vi "Hydrodynamics Method_YCC.vi"(11 "Save?":bool) -> ()   [LabVIEW 2014]
uses:
  <vilib>/Analysis/3filter.llb/Savitzky-Golay Filter (DBL).vi
  <vilib>/DAQmx/create/channels.llb/DAQmx Create Channel (AI-Voltage-Basic).vi
  <vilib>/DAQmx/configure/timing.llb/DAQmx Timing (Sample Clock).vi
  <vilib>/DAQmx/read.llb/DAQmx Read (Analog 1D DBL 1Chan NSamp).vi
  <vilib>/gmath/NumericalOptimization/Nonlinear Curve Fit LM formula string.vi
  Main-Stage-PI/(Global) Current handle and LaserPower_YCC.vi
  <vilib>/Analysis/NI_AALBase.lvlib
  <vilib>/gmath/NI_Gmath.lvlib
panel:
  out "Filtered data":dbl[](array[numeric])
  in  "Who's Data":enum16{"YCC", "PYW", "LCH", "YYH"}(ring)
  in  "Custum Fs (Hz)":i32
  in  "Sampling Rate Enum (Hz)":T1(ring)=enum."131072"
  out "output array":dbl[](array[numeric])
  in  "Filter?":bool=TRUE
  in  "add record time (s)":dbl
  out "data":dbl[](array[numeric])
  out "lower peak (mV)":dbl
  out "upper peak (mV)":dbl
  out "middle peak (mV)":dbl
  in  "Volumn of glycerol":dbl
  in  "Volumn of water":dbl=1.0
  in  "Temperature (C)":dbl=25.0
  out "best fit parameters":dbl[](array[numeric])
  out "best nonlinear fit counts":dbl[](array[numeric])
  out "QPD (1000X V)":dbl[](array[numeric])
  out "Normalized Counts":dbl[](array[numeric])
  out "dx (nm)":dbl
  out "Histogram: h(x)":i32[](array[numeric])
  in  "Cut second from initial":dbl
  in  "side points":i32=32
  out "Axis":i32
  in  "MultiGaussian Fit?":bool=TRUE
  out "Wait between half period (s)":dbl=0.2
  out "Real Current Commanded position (um)":dbl format="%0.5f"
  out "Trap stiffness (pN/nm)":dbl
  out "Drag Force (pN)":dbl
  out "Conversion factor (V/um)":dbl=1.5
  out "dx (V)":dbl
  out "dx2 (mV)":dbl
  out "dx1 (mV)":dbl
  in  "bead height (um)":dbl=2.0
  out "Upper QPD":dbl
  out "Lower QPD":dbl
  out "Center QPD":dbl
  out "Time":dbl[](array[numeric])
  in  "Tab Control":T2(tab)
  out "Raw XY Graph":cluster{dbl[], "data":dbl[]}(graph)
  out "Filtered XY Graph":cluster{dbl[], "Filtered X":dbl[]}(graph)
  out "Histogram Graph":T3(graph)
  out "XY Graph":T4(graph)
  out "Sampling rate (Hz)":dbl=32000.0 format="%0.2f"
  out "traveling time (s)":dbl
  out "True rate?":bool
  in  "T=X\nF=Y":bool=TRUE
  in  "T= + first\nF=- first":bool
  in  "range  (um)":dbl=10.0 min=0.0 max=100.0 step=0.5 format="%.3f"
  in  "scan rate  (um/s)":dbl=200.0 format="%.3f"
  in  "# of period generate\n(0.5,1,1.5,2...)":dbl=4.0
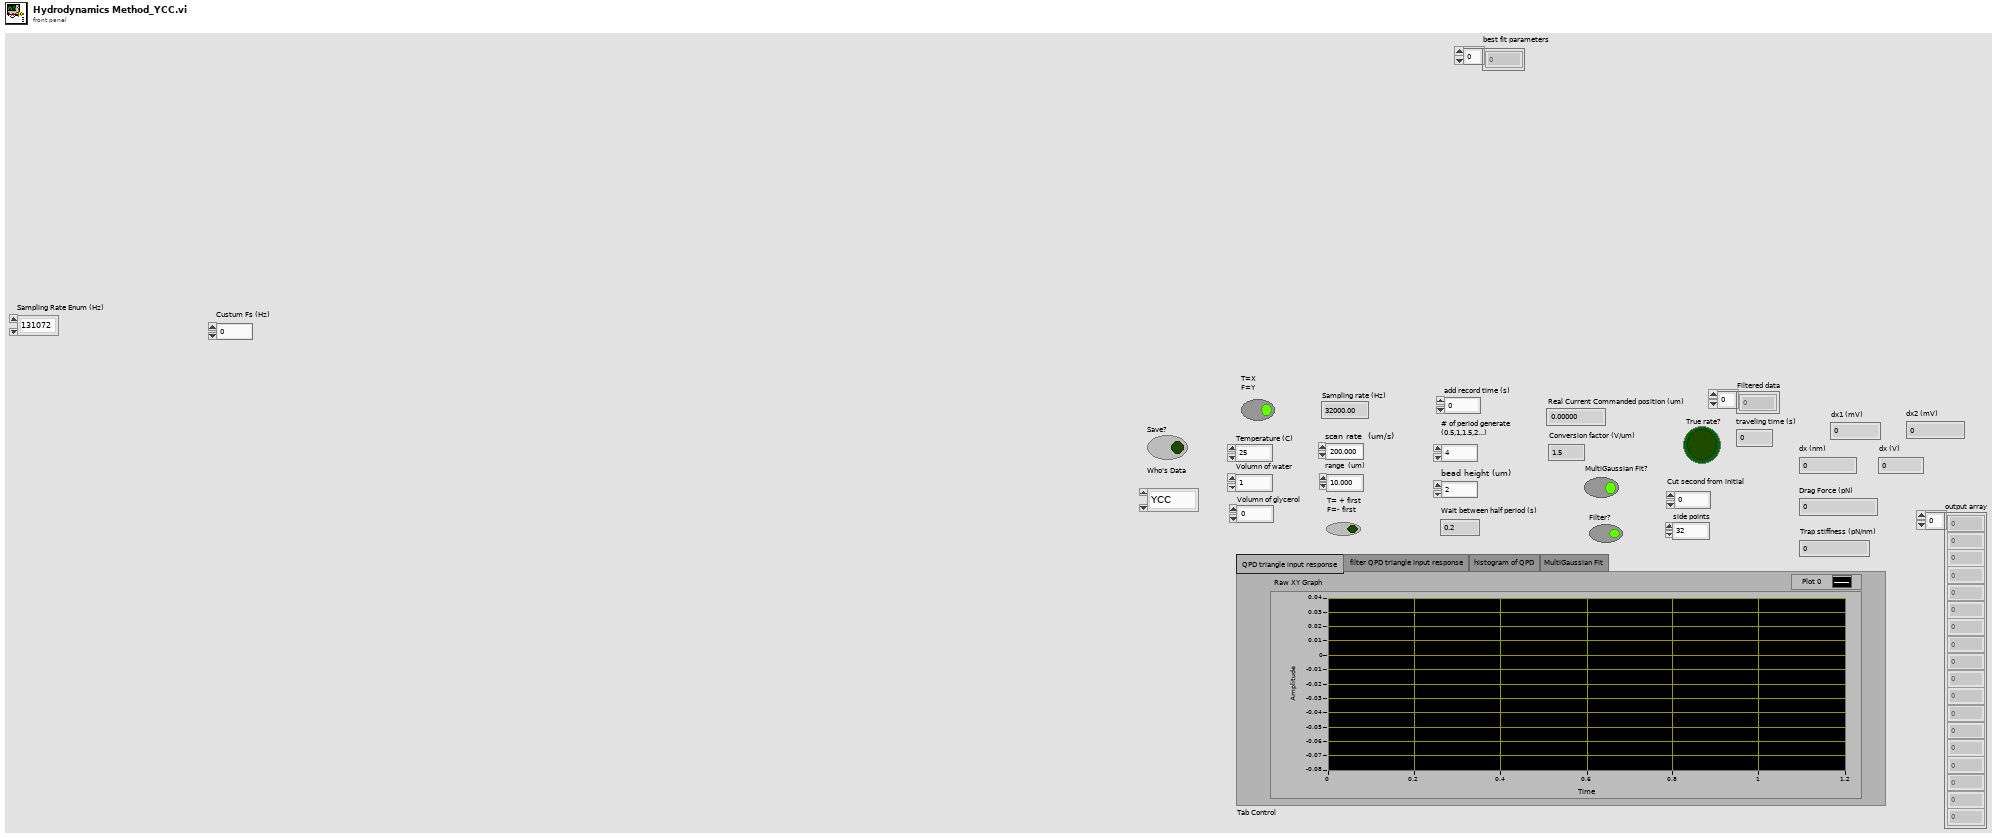
[diagram p1: front panel]
types:
  T1 = enum16{"custum", "16384", "32768", "65536", "131072", "262144"}
  T2 = enum32{"QPD triangle input response ", "filter QPD triangle input response ", "histogram of QPD", "MultiGaussian Fit"}
  T3 = cluster{"X Values":dbl[], "Histogram: h(x)":i32[]}
  T4 = cluster{"QPD (1000X V)":dbl[], "Nor. Counts":dbl[]}[]
  T5 = cluster{"model":string, "Parameters":string[], "x":string}
  T6 = cluster{"QPD (1000X V)":dbl[], "best nonlinear fit counts":dbl[]}
  T7 = cluster{"QPD (1000X V)":dbl[], "Normalized Counts":dbl[]}
  T8 = cluster{"QPD (1000X V)":dbl[], "Normalized Counts":dbl[]}[]
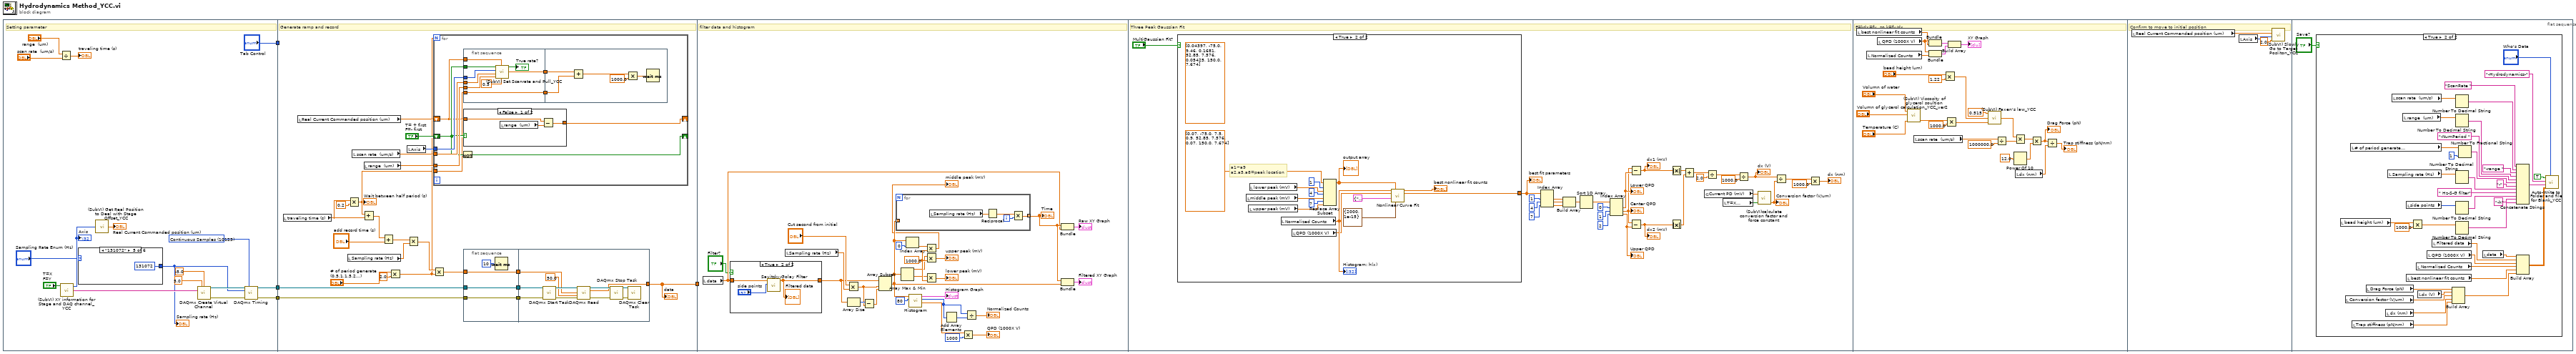
[diagram p0: block diagram]
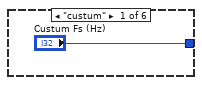
[diagram p2: hidden frame]
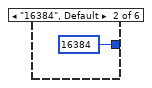
[diagram p3: hidden frame]
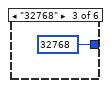
[diagram p4: hidden frame]
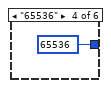
[diagram p5: hidden frame]
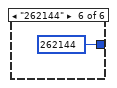
[diagram p6: hidden frame]
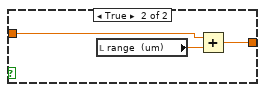
[diagram p7: hidden frame]
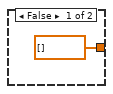
[diagram p9: hidden frame]
diagram:
  n1 = flat-sequence {
    tunnel: ["Tab Control"] -> w4
    tunnel: [w8] -> w2
    tunnel: [w7] -> w1
    tunnel: w4 -> [_]
    tunnel: [w39] -> w3
    tunnel: w2 -> [w43]
    tunnel: w1 -> [w42]
    tunnel: w3 -> [_]
    frame #0 {
      w21 = 10123 items=["Finite Samples"=10178, "Continuous Samples"=10123, "Hardware Timed Single Point"=12522] ("sample mode")
      # "Setting parameter"
      n2 = Divide(x="range  (um)", y="scan rate  (um/s)") -> (x/y=→"traveling time (s)":dbl)
      n3 = call "(SubVI) XY information for Stage and DAQ channel_YCC.vi"("T=X\nF=Y"="T=X\nF=Y") -> ("physical channels"=w17:tag, "Axis"=w10:i32)  [unwired: 3 in]
      "Axis" <- w10
      n4 = case shown="\"131072\"" "Sampling Rate Enum (Hz)" {
        tunnel: ["Custum Fs (Hz)" 16384 32768 65536 131072 262144] -> w5
        frame "custum" {
        }
        frame "16384", Default {
        }
        frame "32768" {
        }
        frame "65536" {
        }
        frame "131072" {
        }
        frame "262144" {
        }
      }
      "Sampling rate (Hz)" <- w5
      n5 = call "(SubVI) Get Real Position to Deal with Stage Offset_YCC.vi"("Axis"=w10) -> ("Real Current Commanded position (um)"=→"Real Current Commanded position (um)":dbl)  [unwired: 3 in, 1 out]
      n6 = call-poly <vilib>:"DAQmx Create Virtual Channel.vi"("maximum value"=5.0, "minimum value"=-5.0, "physical channels"=w17) -> ("task out"=w19:refnum<k21>, "error out"=w20:errorcluster)  [unwired: 6 in, 5 out]
      n7 = call-poly <vilib>:"DAQmx Timing.vi"("task/channels in"=w19, "sample mode"=w21, "rate"=w5, "error in"=w20) -> ("task out"=w8:refnum<k21>, "error out"=w7:errorcluster)  [unwired: 3 in, 7 out]
    }
    frame #1 {
      # "Generate ramp and record"
      n8 = local read "traveling time (s)"() -> (w30:dbl)
      n9 = local read "Real Current Commanded position (um)"() -> (w49:dbl)
      n10 = local read "Sampling rate (Hz)"() -> (w38:dbl)
      n11 = Multiply(x=w30, y=0.2) -> (x*y=w28:dbl)
      "Wait between half period (s)" <- w28
      n12 = local read "scan rate  (um/s)"() -> (w45:dbl)
      n13 = Add(x=w28, y=w30) -> (x+y=w33:dbl)
      n14 = local read "range  (um)"() -> (w46:dbl)
      n15 = Add(x=w33, y="add record time (s)") -> (x+y=w31:dbl)
      n16 = Multiply(x="# of period generate\n(0.5,1,1.5,2...)", y=2.0) -> (x*y=w36:dbl)
      n17 = local read "Axis"() -> (w48:i32)
      n18 = Multiply(x=w31, y=w38) -> (x*y=w37:dbl)
      n19 = Multiply(x=w37, y=w36) -> (x*y=w35:dbl)
      n20 = for {
        N: w36 -> [_]
        shift-right: [w75] -> _
        shift-left: "T= + first\nF=- first" -> [w70]
        tunnel: w48 -> [w74]
        tunnel: w45 -> [w72]
        tunnel: w46 -> [w71]
        shift-right: [w68] -> _
        shift-left: w49 -> [w69]
        tunnel: w28 -> [w66]
        n21 = Not(x=w70) -> (.not. x?=w75:bool)
        n22 = flat-sequence {
          tunnel: w70 -> [w90]
          tunnel: w74 -> [w89]
          tunnel: [w86] -> w73
          tunnel: w72 -> [w85]
          tunnel: w71 -> [w84]
          tunnel: w69 -> [w83]
          tunnel: [w82] -> w67
          tunnel: w66 -> [w82]
          tunnel: w73 -> [w95]
          tunnel: w67 -> [w91]
          frame #0 {
            n23 = call "(SubVI) Set Scanrate and Pull_YCC.vi"("toward+ ?\nT=+, F=-"=w90, "Start From  (um)"=w83, "axis"=w89, "scan rate  (um/s)"=w85, "waiting time per point (ms)\nrange from 5ms to 0.167 ms"=0.5 ("waiting time per point (ms)\nrange from 5ms to 0.167 ms"), "range  (um)"=w84) -> ("True rate?"=→"True rate?":bool, "traveling time (s)"=w86:dbl)  [unwired: 1 out]
          }
          frame #1 {
            n24 = Add(x=w95, y=w91) -> (x+y=w94:dbl)
            n25 = Multiply(x=w94, y=1000.0) -> (x*y=w92:dbl)
            n26 = Wait (ms)(milliseconds to wait=w92) -> ()  [unwired: 1 out]
          }
        }
        n27 = case shown="False" w70 {
          tunnel: w69 -> [w78 w81]
          tunnel: [w76 w79] -> w68
          frame False {
            n28 = local read "range  (um)"() -> (w77:dbl)
            n29 = Subtract(x=w78, y=w77) -> (x-y=w76:dbl)
          }
          frame True {
            n30 = local read "range  (um)"() -> (w80:dbl)
            n31 = Add(x=w81, y=w80) -> (x+y=w79:dbl)
          }
        }
      }
      n32 = flat-sequence {
        tunnel: w42 -> [w53]
        tunnel: w43 -> [w54]
        tunnel: [w54] -> w41
        tunnel: [w53] -> w40
        tunnel: w35 -> [w51]
        tunnel: [w51] -> w34
        tunnel: w41 -> [w65]
        tunnel: w40 -> [w64]
        tunnel: [w57] -> w39
        tunnel: w34 -> [w55]
        frame #0 {
          n33 = Wait (ms)(milliseconds to wait=u32 10) -> ()  [unwired: 1 out]
        }
        frame #1 {
          n34 = call <vilib>:"DAQmx Start Task.vi"("task/channels in"=w65, "error in"=w64) -> ("task out"=w63:refnum<k21>, "error out"=w62:errorcluster)  [unwired: 12 out]
          n35 = call-poly <vilib>:"DAQmx Read.vi"("task/channels in"=w63, "number of samples per channel"=w55, "timeout"=50.0, "error in"=w62) -> ("task out"=w61:refnum<k21>, "data"=w57:dbl[], "error out"=w59:errorcluster)  [unwired: 9 out]
          n36 = call <vilib>:"DAQmx Stop Task.vi"("task/channels in"=w61, "error in"=w59) -> ("task out"=w60:refnum<k21>, "error out"=w58:errorcluster)  [unwired: 12 in]
          n37 = call <vilib>:"DAQmx Clear Task.vi"("task in"=w60, "error in"=w58) -> ()  [unwired: 13 in, 1 out]
        }
      }
      "data" <- w39
    }
    frame #2 {
      w110 = 1000.0 ("y")
      # "filter data and histogram"
      n38 = local read "data"() -> (w98:dbl[])
      n39 = case shown="True" "Filter?" {
        tunnel: [w124 w125] -> w96
        tunnel: w98 -> [w124 w126]
        frame False {
        }
        frame True {
          n40 = call-poly <vilib>:"Savitzky-Golay Filter.vi"("side points"="side points", "X"=w126) -> ("Filtered X"=w125:dbl[])  [unwired: 8 in, 1 out]
          "Filtered data" <- w125
        }
      }
      n41 = local read "Sampling rate (Hz)"() -> (w117:dbl)
      n42 = Multiply(x="Cut second from initial", y=w117) -> (x*y=w115:dbl)
      n43 = Array Size(array=w96) -> (size(s)=w116:i32)
      n44 = Subtract(x=w116, y=w115) -> (x-y=w114:dbl)
      n45 = Array Subset(array=w96, index=w115, length=w114) -> (w112:dbl[])
      n46 = for {
        tunnel: [w128] -> w122 mode=indexing
        tunnel: w112 -> [_] mode=indexing
        i -> [w131]
        n47 = local read "Sampling rate (Hz)"() -> (w130:dbl)
        n48 = Reciprocal(x=w130) -> (1/x=w129:dbl)
        n49 = Multiply(x=w129, y=w131) -> (x*y=w128:dbl)
      }
      "Time" <- w122
      n50 = Array Max & Min(array=w112) -> (max value=w108:dbl, min value=w109:dbl)  [unwired: 2 out]
      n51 = Index Array(array=w112, index=0) -> (element=w111:dbl)
      n52 = call <vilib>:"Histogram.vi"("intervals"=80, "X"=w112) -> ("X Values"=w105:dbl[], "Histogram: h(x)"=w106:i32[], "Histogram Graph"=→"Histogram Graph":T3)  [unwired: 6 in, 1 out]
      n53 = Multiply(x=w111, y=w110) -> (x*y=→"middle peak (mV)":dbl)
      n54 = Multiply(x=w108, y=w110) -> (x*y=→"upper peak (mV)":dbl)
      n55 = Multiply(x=w109, y=w110) -> (x*y=→"lower peak (mV)":dbl)
      n56 = Add Array Elements(numeric array=w106) -> (sum=w107:i32)
      n57 = Multiply(x=w105, y=1000) -> (x*y=→"QPD (1000X V)":dbl[])
      n58 = Divide(x=w106, y=w107) -> (x/y=→"Normalized Counts":dbl[])
      n59 = Bundle(w122, "data"=w98) -> (→"Raw XY Graph":cluster{dbl[], "data":dbl[]})  [unwired: 1 in]
      n60 = Bundle(w122, w112) -> (→"Filtered XY Graph":cluster{dbl[], dbl[]})  [unwired: 1 in]
    }
    frame #3 {
      # "Three Peak Gaussian Fit"
      n61 = case shown="True" "MultiGaussian Fit?" {
        tunnel: [dbl[] [] ("best nonlinear fit") w170] -> w162
        frame False {
        }
        frame True {
          (unwired) dbl[] [0.04397, -75.0, 9.46, 0.1681, 52.85, 7.576, 0.05425, 150.0, 7.674] ("initial parameters")
          # "a1~a9\na2,a5,a8=peak location"
          n62 = local read "middle peak (mV)"() -> (w168:dbl)
          n63 = local read "upper peak (mV)"() -> (w165:dbl)
          n64 = local read "lower peak (mV)"() -> (w164:dbl)
          n65 = local read "Normalized Counts"() -> (w167:dbl[])
          "Histogram: h(x)" <- w167
          n66 = local read "QPD (1000X V)"() -> (w166:dbl[])
          n67 = Replace Array Subset(array=dbl[] [0.07, -75.0, 7.5, 0.9, 52.85, 7.576, 0.07, 150.0, 7.674] ("initial parameters"), new element #1=w164, index #1=1 ("index"), new element #2=w168, index #2=4 ("index"), new element #3=w165, index #3=7 ("index")) -> (w171:dbl[])
          "output array" <- w171
          n68 = call-poly <vilib>:"Nonlinear Curve Fit.vi"("Y"=w167, "initial parameters"=w171, "X"=w166, "model description"=T5 {"model"="a1*exp(-((u-a2)/a3)^2)+a4*exp(-((u-a5)/a6)^2)+a7*exp(-((u-a8)/a9)^2)", "Parameters"=["a1", "a2", "a3", "a4", "a5", "a6", "a7", "a8", "a9"], "x"="u"}, "termination"=cluster{"max iteration":i32, "tolerance":dbl} {"max iteration"=2000, "tolerance"=1e-15}) -> ("best nonlinear fit"=→"best nonlinear fit counts":dbl[], "best fit parameters"=w170:dbl[])  [unwired: 6 in, 3 out]
        }
      }
      "best fit parameters" <- w162
      n69 = Index Array(array=w162, index #1=1 ("index"), index #2=4 ("index"), index #3=7 ("index")) -> (element #1=w158:dbl, element #2=w157:dbl, element #3=w156:dbl)
      n70 = Build Array(w158, w157, w156) -> (w155:dbl[])
      n71 = Sort 1D Array(array=w155) -> (sorted array=w154:dbl[])
      n72 = Index Array(array=w154, index #1=0 ("index"), index #2=1 ("index"), index #3=2 ("index")) -> (element #1=w150:dbl, element #2=w133:dbl, element #3=w132:dbl)
      "Center QPD" <- w133
      "Lower QPD" <- w150
      "Upper QPD" <- w132
      n73 = Subtract(x=w133, y=w150) -> (x-y=w134:dbl)
      "dx1 (mV)" <- w134
      n74 = Subtract(x=w133, y=w132) -> (x-y=w135:dbl)
      "dx2 (mV)" <- w135
      n75 = Absolute Value(x=w134) -> (abs(x)=w149:dbl)
      n76 = Absolute Value(x=w135) -> (abs(x)=w148:dbl)
      n77 = Add(x=w149, y=w148) -> (x+y=w147:dbl)
      n78 = global read "(Global) Current handle and LaserPower_YCC.vi" "Current PD (mV)"() -> (w140:dbl)
      n79 = Divide(x=w147, y=2.0) -> (x/y=w144:dbl)
      n80 = local read "T=X\nF=Y"() -> (w141:bool)
      n81 = Divide(x=w144, y=1000.0) -> (x/y=w142:dbl)
      "dx (V)" <- w142
      n82 = call "(SubVI)calculate conversion factor and force constant.vi"("X=T\nY=F"=w141, "laser power (mW)"=w140) -> ("conversion factor (V/um)"=w139:dbl)  [unwired: 2 in, 1 out]
      "Conversion factor (V/um)" <- w139
      n83 = Divide(x=w142, y=w139) -> (x/y=w136:dbl)
      n84 = Multiply(x=w136, y=1000.0) -> (x*y=→"dx (nm)":dbl)
    }
    frame #4 {
      # "F=kdx=fv  so k=fv/dx"
      n85 = local read "best nonlinear fit counts"() -> (w194:dbl[])
      n86 = local read "Normalized Counts"() -> (w195:dbl[])
      n87 = local read "QPD (1000X V)"() -> (w196:dbl[])
      n88 = call "(SubVI) Viscosity of glycerol soultion calculation_YCC_ver2.vi"("Volumn of water"="Volumn of water", "Volumn of glycerol"="Volumn of glycerol", "Temperature (C)"="Temperature (C)") -> ("Viscosity of mix (Pa*s)"=w184:dbl)  [unwired: 4 in, 1 out]
      n89 = local read "scan rate  (um/s)"() -> (w190:dbl)
      n90 = Bundle("QPD (1000X V)"=w196, "best nonlinear fit counts"=w194) -> (w193:T6)  [unwired: 1 in]
      n91 = Bundle("QPD (1000X V)"=w196, "Normalized Counts"=w195) -> (w192:T7)  [unwired: 1 in]
      n92 = Multiply(x="bead height (um)", y=1.22 ("Focal shift factor")) -> (x*y=w185:dbl)
      n93 = Multiply(x=w184, y=1000.0) -> (x*y=w182:dbl)
      n94 = Build Array(w193, w192) -> (→"XY Graph":T8)
      n95 = call "(SubVI) Faxen's law_YCC.vi"("viscosity (cP)"=w182, "bead height (um)"=w185, "bead radius (um)"=0.515) -> ("Faxen's law of friction coefficient (N/(m/s))"=w202:dbl)  [unwired: 2 in]
      n96 = Divide(x=w190, y=1000000.0) -> (x/y=w188:dbl)
      n97 = Multiply(x=w202, y=w188) -> (x*y=w201:dbl)
      n98 = Power Of 10(x=12.0) -> (10^x=w199:dbl)
      n99 = local read "dx (nm)"() -> (w178:dbl)
      n100 = Multiply(x=w201, y=w199) -> (x*y=w197:dbl)
      "Drag Force (pN)" <- w197
      n101 = Divide(x=w197, y=w178) -> (x/y=→"Trap stiffness (pN/nm)":dbl)
    }
    frame #5 {
      # "Confirm to move to initial position"
      n102 = local read "Real Current Commanded position (um)"() -> (w206:dbl)
      n103 = local read "Axis"() -> (w205:i32)
      n104 = call "(SubVI) Slowly Go to Target Posiiton_YCC.vi"("scan rate  (um/s)"=2.0, "axis"=w205, "Target position (um)"=w206) -> ()  [unwired: 1 in, 4 out]
    }
    frame #6 {
      n105 = case shown="True" "Save?" {
        frame False {
        }
        frame True {
          n106 = local read "bead height (um)"() -> (w236:dbl)
          n107 = local read "Conversion factor (V/um)"() -> (w212:dbl)
          n108 = local read "# of period generate\n(0.5,1,1.5,2...)"() -> (w223:dbl)
          n109 = local read "Trap stiffness (pN/nm)"() -> (w210:dbl)
          n110 = local read "Drag Force (pN)"() -> (w214:dbl)
          n111 = local read "dx (nm)"() -> (w211:dbl)
          n112 = local read "Sampling rate (Hz)"() -> (w233:dbl)
          n113 = local read "scan rate  (um/s)"() -> (w232:dbl)
          n114 = local read "range  (um)"() -> (w231:dbl)
          n115 = local read "side points"() -> (w237:i32)
          n116 = local read "best nonlinear fit counts"() -> (w215:dbl[])
          n117 = Multiply(x=w236, y=1000.0) -> (x*y=w234:dbl)
          n118 = local read "Normalized Counts"() -> (w216:dbl[])
          n119 = local read "dx (V)"() -> (w213:dbl)
          n120 = local read "QPD (1000X V)"() -> (w217:dbl[])
          n121 = local read "Filtered data"() -> (w218:dbl[])
          n122 = Build Array(w214, w213, w212, w211, w210) -> (w209:dbl[])
          n123 = Number To Decimal String(number=w232) -> (decimal integer string=w229:string)  [unwired: 1 in]
          n124 = Number To Decimal String(number=w231) -> (decimal integer string=w227:string)  [unwired: 1 in]
          n125 = Number To Decimal String(number=w233) -> (decimal integer string=w224:string)  [unwired: 1 in]
          n126 = Number To Decimal String(number=w237) -> (decimal integer string=w240:string)  [unwired: 1 in]
          n127 = Number To Decimal String(number=w234) -> (decimal integer string=w239:string)  [unwired: 1 in]
          n128 = Number To Fractional String(number=w223, precision (6)=i16 1) -> (F-format string=w220:string)  [unwired: 2 in]
          n129 = local read "data"() -> (w225:dbl[])
          n130 = Concatenate Strings("ScanRate " ("string"), w229, "-range " ("string"), w227, "-NumPeriod " ("string"), w220, "-" ("string"), w224, " Hz-S-G filter" ("string"), w240, "-h" ("string"), w239) -> (w226:string)
          n131 = Build Array(w225, w218, w217, w216, w215, w209) -> (w208:dbl[][])
          n132 = call "Auto-Write to Folder and file for Blank_YCC.vi"("Who's Data"="Who's Data", "data to be saved"=w208, "File name add to the end \n(height)"=w226, "Title"="-Hydrodynamics-", "Save?"=TRUE) -> ()  [unwired: 3 in, 2 out]
        }
      }
    }
  }
